vi "Spin Wheels.vi"(8 "error in (no error)":errorcluster, 9 "Right Wheel Power":dbl, 10 "Left Wheel Power":dbl, 11 "Dev Grabber in":refnum<class "Dev Grabber.lvclass">) -> (0 "error out":errorcluster, 3 "Dev Grabber out":refnum<class "Dev Grabber.lvclass">)   [LabVIEW 2014, in "Dev Grabber.lvlib" / "Dev Grabber.lvclass"]
uses:
  Dev Grabber.lvclass
  Dev Grabber.lvclass/Dev Grabber.ctl
  Robot/Grabber/Grabber Class/Grabber.lvclass
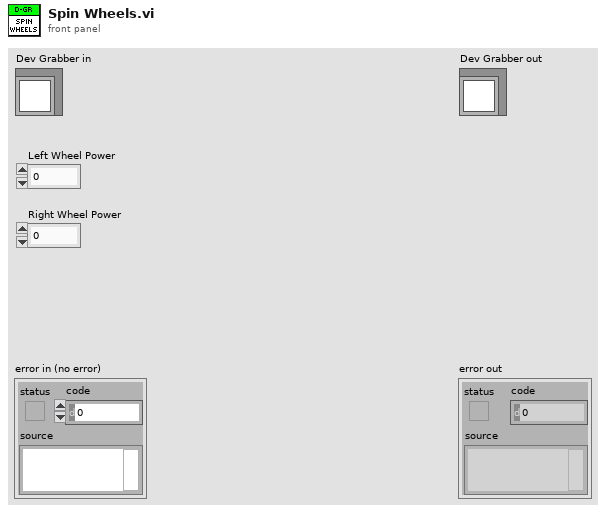
[diagram p1: front panel]
types:
  T1 = typedef "WPI_MotorControlDeviceRef.ctl" = cluster{"DeviceStatus":errorcluster, "Type":T2, "PWM":cluster{"Controller":T3, "PWM Channel":T4, "DeadBand":T5}, "CAN":cluster{"Device Number":u8, "Control Mode":T6, "Semaphore":T7, "Max Vout":dbl, "TalonSRX Control Mode":T8}, "Invert":bool, "TransformRef":T9, "InvTransformRef":T9}
  T2 = typedef "WPI_MotorControlType.ctl" = enum16{"PWM", "CAN", "CANTalonSRX"}
  T3 = typedef "FPGA_TypedefDigitalModule.ctl" = enum16{"Controller 1"}
  T4 = typedef "FPGA_DIOPWMChannel.ctl" = enum8{"PWM 0", "PWM 1", "PWM 2", "PWM 3", "PWM 4", "PWM 5", "PWM 6", "PWM 7", "PWM 8", "PWM 9", "PWM MXP 0", "PWM MXP 1", "PWM MXP 2", "PWM MXP 3", "PWM MXP 4", "PWM MXP 5", "PWM MXP 6", "PWM MXP 7", "PWM MXP 8", "PWM MXP 9", "Invalid"}
  T5 = typedef "WPI_PWMDeadband.ctl" = cluster{"Name":string, "maxPositivePwm":i32, "minPositivePwm":i32, "centerPwm":i32, "maxNegativePwm":i32, "minNegativePwm":i32, "angularRange":u16}
  T6 = typedef "WPI_CANJaguar_ControlMode.ctl" = enum8{"Percent VBus", "Current", "Speed", "Position", "Voltage"}
  T7 = typedef "Semaphore RefNum" = refnum<k1>
  T8 = typedef "WPI_CANTalonSRX_APIControlMode.ctl" = enum8{"Percent VBus", "Speed", "Position", "Slave", "Unchanged / Invalid"}
  T9 = typedef "WPI_PWMTransform_ConPane.ctl" = refnum<vi>
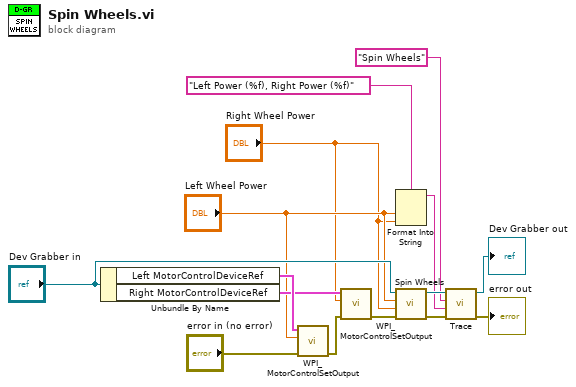
[diagram p0: block diagram]
diagram:
  n1 = Unbundle By Name("Dev Grabber in") -> ("Left MotorControlDeviceRef"=w14:T1, "Right MotorControlDeviceRef"=w13:T1)
  n2 = call <vilib>:"WPI_MotorControlSetOutput.vi"("error in (no error)"="error in (no error)", "Output"="Left Wheel Power", "MotorControlDevRef"=w14) -> ("error out"=w11:errorcluster)  [unwired: 6 in, 2 out]
  n3 = call <vilib>:"WPI_MotorControlSetOutput.vi"("error in (no error)"=w11, "Output"="Right Wheel Power", "MotorControlDevRef"=w13) -> ("error out"=w10:errorcluster)  [unwired: 6 in, 2 out]
  n4 = Format Into String(format string="Left Power (%f), Right Power (%f)", "Left Wheel Power", "Right Wheel Power") -> (resulting string=w3:string)  [unwired: 2 in, 1 out]
  n5 = call-parent "Spin Wheels.vi"("error in (no error)"=w10, "Right Wheel Power"="Right Wheel Power", "Left Wheel Power"="Left Wheel Power", "Grabber in"="Dev Grabber in") -> ("error out"=w9:errorcluster, "Grabber out"=w8:refnum<class "Dev Grabber.lvclass">)  [unwired: 6 in]
  n6 = call-dynamic "Trace.vi"("error in (no error)"=w9, "System Message"=w3, "System Action"="Spin Wheels", "System Actor in"=w8) -> ("error out"=→"error out":errorcluster, "System Actor out"=→"Dev Grabber out":refnum<class "Dev Grabber.lvclass">)  [unwired: 6 in]
